vi "07TRM800_GetScopegraph.vi"() -> ()   [LabVIEW 2015]
panel:
  out "Waveform Graph":i8[](graph)
  out "length":i32
  out "size(s)":i32
  out "String":string
  out "Array":u16[](array[numeric])
  out "element":bool
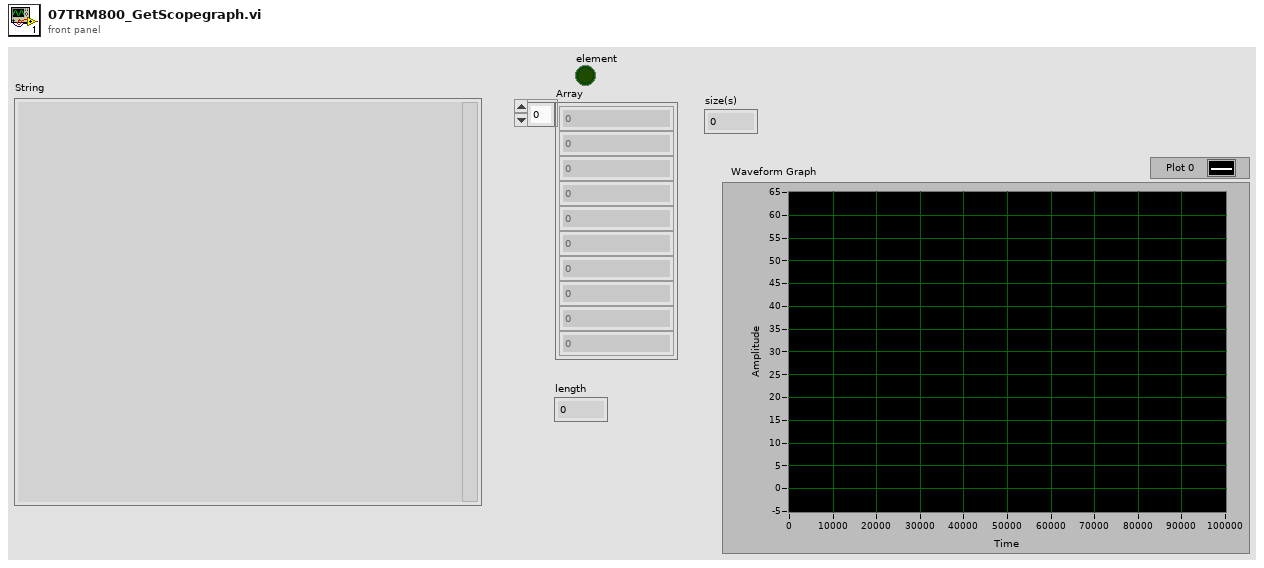
[diagram p1: front panel]
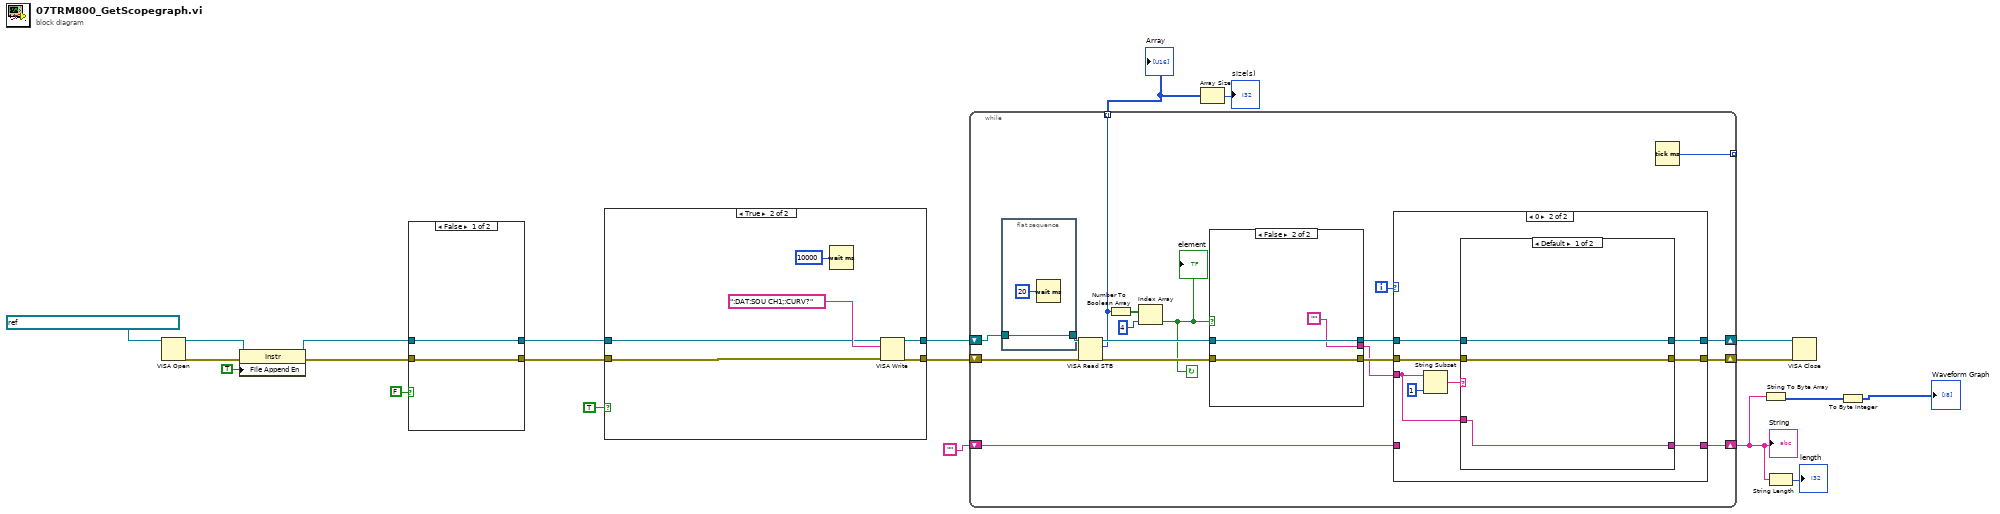
[diagram p0: block diagram]
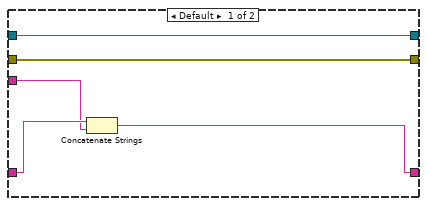
[diagram p3: hidden frame]
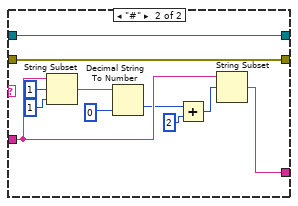
[diagram p4: hidden frame]
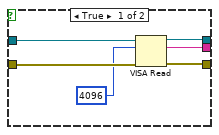
[diagram p5: hidden frame]
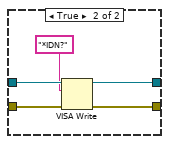
[diagram p6: hidden frame]
diagram:
  n1 = VISA Open(VISA resource name=refnum<visa-resource-name> "USB0::0x0699::0x03A3::C030457::INSTR") -> (VISA resource name=w11:refnum<visa-resource-name>, error out=w12:errorcluster)  [unwired: 4 in]
  n2 = property class="Instr"(reference=w11, error in=w12, "File Append En"=TRUE ("Message Based Settings:File Append Enable")) -> (reference out=w10:refnum<visa-resource-name>, error out=w9:errorcluster)
  n3 = case shown="False" FALSE {
    tunnel: [w23 w26] -> w17
    tunnel: w10 -> [w23 w28]
    tunnel: [w22 w25] -> w16
    tunnel: w9 -> [w22 w27]
    frame False {
    }
    frame True {
      n4 = VISA Write(VISA resource name=w28, write buffer="*IDN?", error in (no error)=w27) -> (VISA resource name out=w26:refnum<visa-resource-name>, error out=w25:errorcluster)  [unwired: 1 out]
    }
  }
  n5 = case shown="True" TRUE {
    tunnel: w17 -> [w30 w32]
    tunnel: w16 -> [w29 w31]
    tunnel: [w30 w34] -> w15
    tunnel: [w29 w35] -> w14
    frame False {
    }
    frame True {
      n6 = Wait (ms)(milliseconds to wait=u32 10000) -> ()  [unwired: 1 out]
      n7 = VISA Write(VISA resource name=w32, write buffer=":DAT:SOU CH1;:CURV?", error in (no error)=w31) -> (VISA resource name out=w34:refnum<visa-resource-name>, error out=w35:errorcluster)  [unwired: 1 out]
    }
  }
  n8 = while {
    shift-right: [w42] -> w19
    shift-left: w15 -> [w47]
    shift-right: [w39] -> w18
    shift-left: w14 -> [w54]
    tunnel: [w46] -> w7 mode=indexing
    shift-right: [w41] -> w3
    shift-left: "" -> [w40]
    tunnel: [w38] -> _ mode=indexing
    i -> [w45]
    stop <- w49 continue-if-true
    n9 = flat-sequence {
      tunnel: [w83] -> w48
      tunnel: w47 -> [w83]
      frame #0 {
        n10 = Wait (ms)(milliseconds to wait=u32 20) -> ()  [unwired: 1 out]
      }
    }
    n11 = VISA Read STB(8:w54, 11:w48) -> (0:w52:errorcluster, 2:w46:u16, 3:w53:refnum<visa-resource-name>)
    n12 = Number To Boolean Array(number=w46) -> (Boolean array=w51:bool[])
    n13 = Index Array(array=w51, index=4) -> (element=w49:bool)
    "element" <- w49
    n14 = case shown="False" w49 {
      tunnel: w53 -> [w88 w92]
      tunnel: w52 -> [w89 w91]
      tunnel: [w86 w92] -> w44
      tunnel: [w85 w91] -> w43
      tunnel: [w84 ""] -> w37
      frame True {
        n15 = VISA Read(VISA resource name=w88, byte count=u32 4096, error in (no error)=w89) -> (VISA resource name out=w86:refnum<visa-resource-name>, read buffer=w84:string, error out=w85:errorcluster)  [unwired: 1 out]
      }
      frame False {
      }
    }
    n16 = case shown="0" w45 {
      tunnel: w44 -> [w59 w65]
      tunnel: w37 -> [w56 w61]
      tunnel: w43 -> [w58 w64]
      tunnel: [w59 w63] -> w42
      tunnel: [w58 w62] -> w39
      tunnel: [w55 w60] -> w41
      tunnel: w40 -> [w57 _]
      frame Default {
        n17 = Concatenate Strings(w57, w56) -> (w55:string)
      }
      frame 0 {
        n18 = String Subset(string=w61, length (rest)=1 ("length (rest)")) -> (substring=w66:string)  [unwired: 1 in]
        n19 = case shown="Default" w66 {
          tunnel: w61 -> [w68 w76]
          tunnel: w65 -> [w70 w77]
          tunnel: w64 -> [w69 w78]
          tunnel: [w70 w77] -> w63
          tunnel: [w69 w78] -> w62
          tunnel: [w68 w71] -> w60
          frame Default {
          }
          frame "#" {
            n20 = String Subset(string=w76, offset (0)=1, length (rest)=1 ("length (rest)")) -> (substring=w79:string)
            n21 = Decimal String To Number(string=w79, default (0L)=0 ("offset (0)")) -> (number=w73:i32)  [unwired: 1 in, 1 out]
            n22 = Add(x=w73, y=2 ("offset (0)")) -> (x+y=w72:i32)
            n23 = String Subset(string=w76, offset (0)=w72) -> (substring=w71:string)  [unwired: 1 in]
          }
        }
      }
    }
    n24 = Tick Count (ms)() -> (millisecond timer value=w38:u32)
  }
  "Array" <- w7
  "String" <- w3
  n25 = Array Size(array=w7) -> (size(s)=→"size(s)":i32)
  n26 = String To Byte Array(string=w3) -> (unsigned byte array=w2:u8[])
  n27 = String Length(string=w3) -> (length=→"length":i32)
  n28 = VISA Close(VISA resource name=w19, error in (no error)=w18) -> ()  [unwired: 1 out]
  n29 = To Byte Integer(number=w2) -> (8bit integer=→"Waveform Graph":i8[])
